vi "Handle Command.vi"(8 "error in":errorcluster, 10 "Change Laser Vrange in":refnum<class "Change Laser Vrange.lvclass">, 11 "Object In":refnum<class>) -> (0 "error out":errorcluster, 1 "Command Successful?":bool, 2 "Change Laser Vrange Out":refnum<class "Change Laser Vrange.lvclass">, 3 "Object Out":refnum<class>)   [LabVIEW 2014, in "ePAS Library.lvlib" / "Change Laser Vrange.lvclass"]
doc: "Abstract method for accomplishing the execution of a command directed to an instrument object on the wire."
uses:
  Change Laser Vrange.lvclass
  Instrument/ePAS.lvclass
  Instrument/ePAS.lvclass/ePAS.ctl
  Change Laser Vrange.lvclass/Change Laser Vrange.ctl
  reusable/Instrument/Instrument.lvclass/Instrument.ctl
  reusable/Instrument/Read ExtCom.vi
  reusable/Instrument/Read Log Session.vi
  <vilib>/Utility/error.llb/Error Cluster From Error Code.vi
  <vilib>/rvi/errors/niLvFpgaAdjustHostInterfaceError.vi
  <userlib>/_Session Fwk/Session - Root.lvclass
  <vilib>/rvi/interface/nirviReadWriteControl/nirviReadWriteControl.xnode
  FPGA/R FPGA Ref.ctl
  FPGA Bitfiles/FPGAServerV2.lvbitx
  FPGA/Session/Exscalabar FPGA.lvclass
  ePAS Library.lvlib
  reusable/Session APIs/Session Log/System Log.lvclass
  NiFpgaLv.dll
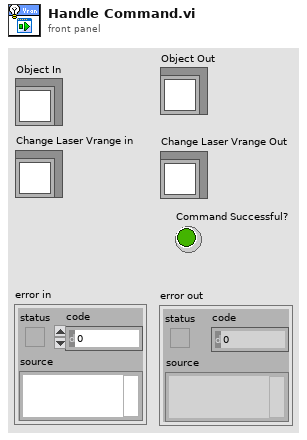
[diagram p1: front panel]
types:
  T1 = typedef "Session - Root.lvclass/Session Handle.ctl" = refnum<data-value>
  T2 = typedef "ePAS Library.lvlib/R FPGA Ref.ctl" = refnum<k20>
  T3 = cluster{"f0":fxp<+,32,0>, "Scale":fxp<+,32,0>, "Offset":i16, "Mod":enum8{"Sine", "Square"}}
  T4 = cluster{"f0":fxp<+,32,0>, "Scale":fxp<+,32,0>, "Offset":i16, "Mod":enum8{"Sine", "Square"}}[]
  T5 = cluster{"tag":string, "section":string, "data":variant}
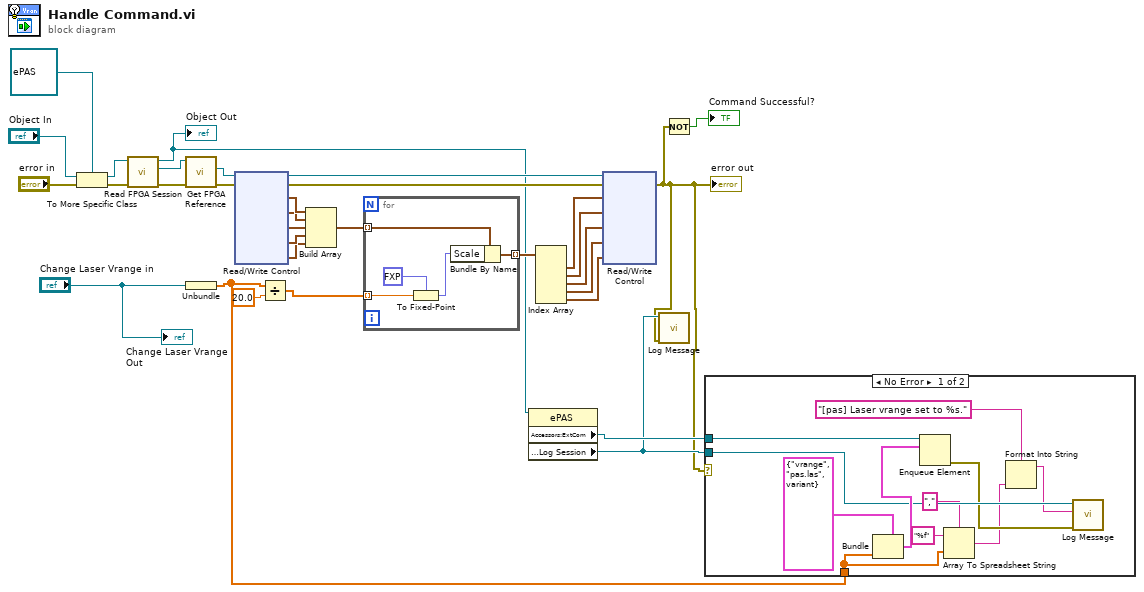
[diagram p0: block diagram]
diagram:
  n1 = To More Specific Class(target class=refnum<class "ePAS.lvclass"> refnum ("ePAS"), reference="Object In", error in="error in") -> (specific class reference=w30:refnum<class "ePAS.lvclass">, error out=w29:errorcluster)
  n2 = call "Read FPGA Session.vi"("error in (no error)"=w29, "ePAS in"=w30) -> ("error out"=w12:errorcluster, "Session Handle"=w28:T1, "ePAS out"=w4:refnum<class "ePAS.lvclass">)  [unwired: 7 in]
  "Object Out" <- w4
  n3 = call "Get FPGA Reference.vi"("error in"=w12, "Session In"=w28) -> ("error out"=w10:errorcluster, "Ex FPGA Ref"=w27:T2)  [unwired: 7 in, 1 out]
  n4 = Unbundle("Change Laser Vrange in") -> (w5:dbl[])
  n5 = xnode "Read/Write Control"("FPGA VI Reference In"=w27, "error in"=w10) -> ("FPGA VI Reference Out"=w20:T2, "error out"=w19:errorcluster, "Cell 1"=w26:T3, "Cell 2"=w25:T3, "Cell 3"=w24:T3, "Cell 4"=w23:T3, "Cell 5"=w22:T3)
  n6 = Divide(x=w5, y=20.0) -> (x/y=w8:dbl[])
  n7 = Build Array(w26, w25, w24, w23, w22) -> (w21:T4)
  n8 = for {
    tunnel: w21 -> [w37] mode=indexing
    tunnel: w8 -> [w36] mode=indexing
    tunnel: [w33] -> w18 mode=indexing
    n9 = To Fixed-Point(fixed-point type=fxp<+,32,0> 0.0 ("f0"), number=w36) -> (fixed-point=w34:fxp<+,32,0>)
    n10 = Bundle By Name(cluster=w37, "Scale"=w34) -> (w33:T3)
  }
  n11 = property class="ePAS"(reference=w4) -> ("Accessors:ExtCom"=w3:refnum<queue>, "Accessors:Log Session"=w2:T1)  [unwired: 1 in, 2 out]
  n12 = Index Array(array=w18) -> (element #1=w17:T3, element #2=w16:T3, element #3=w15:T3, element #4=w14:T3, element #5=w13:T3)  [unwired: 5 in]
  n13 = xnode "Read/Write Control"("FPGA VI Reference In"=w20, "error in"=w19, "Cell 1"=w17, "Cell 2"=w16, "Cell 3"=w15, "Cell 4"=w14, "Cell 5"=w13) -> ("error out"=w1:errorcluster)  [unwired: 1 out]
  "error out" <- w1
  n14 = call "Log Message.vi"("error in"=w1, "session in"=w2) -> ()  [unwired: 8 in, 2 out]
  n15 = Not(x=w1) -> (.not. x?=→"Command Successful?":bool)
  n16 = case shown="No Error" w1 {
    tunnel: w3 -> [w48 _]
    tunnel: w5 -> [w41 _]
    tunnel: w2 -> [w45 _]
    frame No Error {
      n17 = Bundle(cluster=T5 {"tag"="vrange", "section"="pas.las", "data"=variant} ("element"), "data"=w41) -> (w46:T5)  [unwired: 2 in]
      n18 = Enqueue Element(queue=w48, element=w46) -> (error out=w42:errorcluster)  [unwired: 2 in, 2 out]
      n19 = Array To Spreadsheet String(delimiter (Tab)=",", array=w41, 3:"%f" ("format string")) -> (spreadsheet string=w39:string)
      n20 = Format Into String(format string="[pas] Laser vrange set to %s.", w39) -> (resulting string=w43:string)  [unwired: 2 in, 1 out]
      n21 = call "Log Message.vi"("error in"=w42, "MSG In"=w43, "session in"=w45) -> ()  [unwired: 7 in, 2 out]
    }
    frame Error {
    }
  }
  "Change Laser Vrange Out" <- "Change Laser Vrange in"
